vi "sub_数组收尾行对调.vi"(1 "Pulse Number":enum16{"SP", "DP"}(ring)=enum."DP", 2 "Input":i16[][](array[numeric])) -> (0 "output":i16[][](array[numeric]))   [LabVIEW 2015]
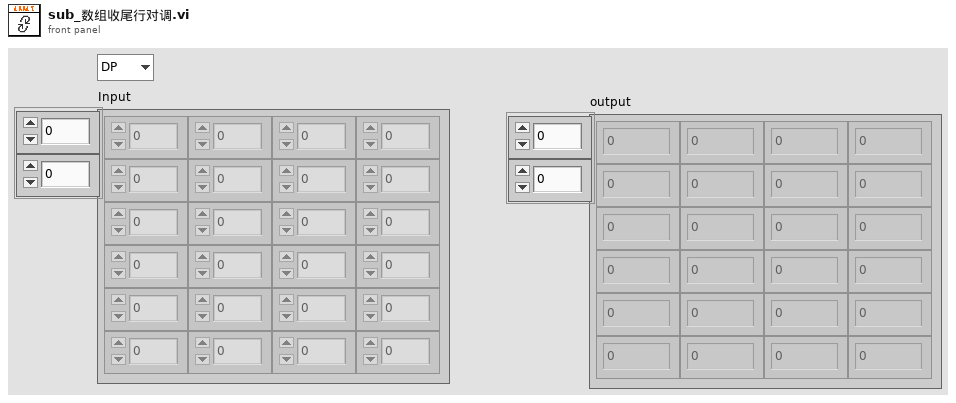
[diagram p1: front panel]
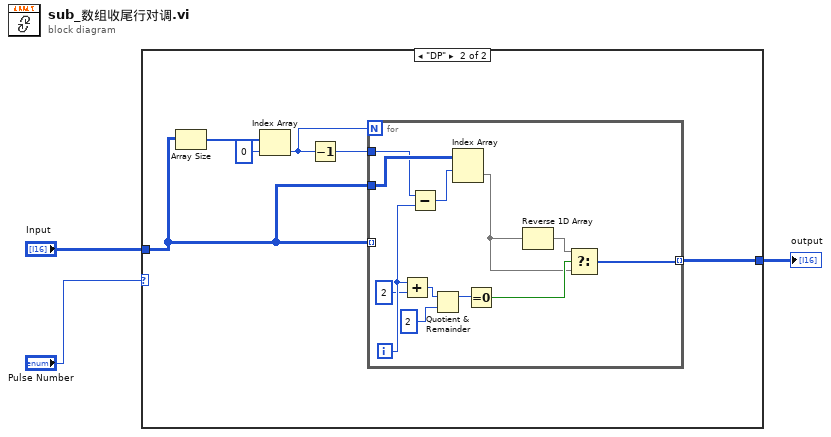
[diagram p0: block diagram]
diagram:
  n1 = case shown="\"DP\"" "Pulse Number" {
    tunnel: "Input" -> [w4 w7]
    tunnel: [w4 w8] -> w2
    frame "SP", Default {
    }
    frame "DP" {
      n2 = Array Size(array=w7) -> (size(s)=w9:i32[])
      n3 = Index Array(array=w9, index=0 ("索引")) -> (element=w6:i32)
      n4 = Decrement(x=w6) -> (x-1=w5:i32)
      n5 = for {
        N: w6 -> [_]
        tunnel: w7 -> [_] mode=indexing
        tunnel: [w18] -> w8 mode=indexing
        tunnel: w7 -> [w17]
        tunnel: w5 -> [w16]
        i -> [w13]
        n6 = Add(x=w13, y=2) -> (x+y=w11:i32)
        n7 = Subtract(x=w16, y=w13) -> (x-y=w15:i32)
        n8 = Quotient & Remainder(x=w11, y=2) -> (x-y*floor(x/y)=w21:i32)  [unwired: 1 out]
        n9 = Index Array(array=w17, index (row)=w15) -> (element=w14:i16[])  [unwired: 1 in]
        n10 = Equal To 0?(x=w21) -> (x = 0?=w19:bool)
        n11 = Reverse 1D Array(array=w14) -> (reversed array=w20:i16[])
        n12 = Select(t=w20, s=w19, f=w14) -> (s? t:f=w18:i16[])
      }
    }
  }
  "output" <- w2
